vi "Guardar_Datos_v2.vi"(0 "File Path Control":path, 1 "Min_Array":dbl[](array[numeric]), 2 "Append/New??":bool, 3 "# Dato IN":u32, 5 "Error In":errorcluster) -> (14 "# Dato Out":u32, 19 "Error Out":errorcluster)   [LabVIEW 2013]
uses:
  <vilib>/Utility/file.llb/Write To Spreadsheet File (DBL).vi
  <vilib>/Analysis/Matrix/NI_Matrix.lvlib
  <vilib>/Analysis/Matrix/Numeric/Conversions/Array To Matrix - RA2.vi
panel:
  # "False =NEW"
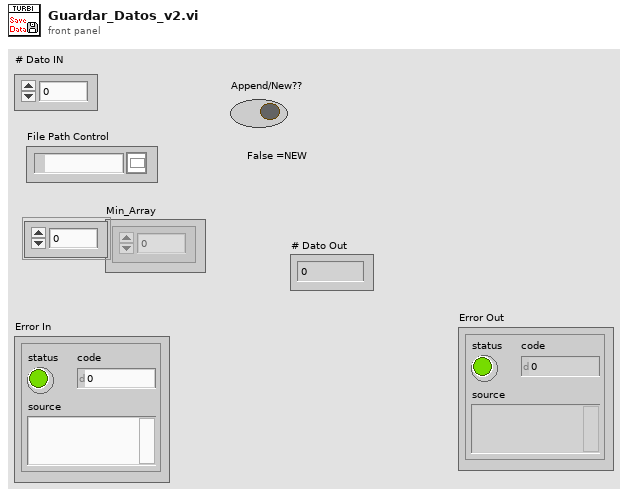
[diagram p1: front panel]
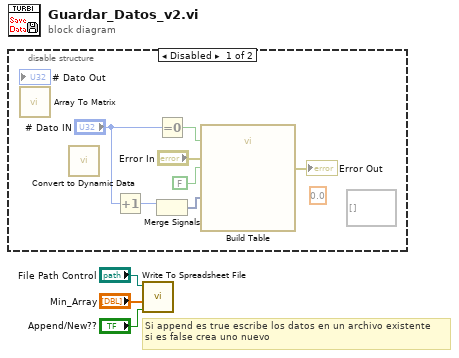
[diagram p0: block diagram]
diagram:
  # "Si append es true escribe los datos en un archivo existente\nsi es false crea uno nuevo"
  n1 = disable-structure shown="Disabled" {
    frame Disabled {
      (unwired) void[][] [] ("Real 2D Array")
      (unwired) 0.0 ("Real Matrix Element")
      n2 = call-poly <vilib>:"Array To Matrix.vi"() -> ()  [unwired: 1 in, 1 out]
      n3 = call "Convert to Dynamic Data"() -> ()  [unwired: 4 in, 1 out]
      n4 = Increment(x="# Dato IN") -> (x+1=w8:u32)
      n5 = Equal To 0?(x="# Dato IN") -> (x = 0?=w6:bool)
      n6 = Merge Signals(w8) -> (w7:dynamicdata)  [unwired: 1 in]
      n7 = call "Build Table"("Include time data"=FALSE, "error in (no error)"="Error In", "Reset"=w6, "Signals"=w7) -> ("error out"=→"Error Out":errorcluster)  [unwired: 1 in, 6 out]
    }
    frame Enabled {
    }
  }
  n8 = call-poly <vilib>:"Write To Spreadsheet File.vi"("append to file? (new file:F)"="Append/New??", "1D data"="Min_Array", "file path (dialog if empty)"="File Path Control") -> ()  [unwired: 5 in, 1 out]
